vi "DiscArchiver.get library version.vi"() -> (0 "nameAndVersion":string)   [LabVIEW 2014, in "DiscArchiver.lvlib"]
doc: "obtain name and version of a library as a string"
uses:
  DiscArchiver.lvlib
  CSlibraries/UtilityLib/UtilityLib.lvlib
  DataLib/DataLib.lvlib
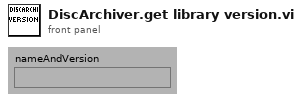
[diagram p1: front panel]
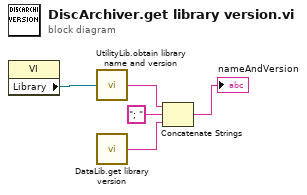
[diagram p0: block diagram]
diagram:
  n1 = property class="VI"() -> ("Library"=w5:refnum<vi>)  [unwired: 2 in, 2 out]
  n2 = call "UtilityLib.obtain library name and version.vi"("Library"=w5) -> ("nameAndVersion"=w4:string)
  n3 = call "DataLib.get library version.vi"() -> ("nameAndVersion"=w3:string)  [unwired: 1 in]
  n4 = Concatenate Strings(w4, "; " ("string"), w3) -> (→"nameAndVersion":string)
